vi "Compile - Buffered Tx Channel Refs.vi"(6 "Packet Name":string, 7 "Timestamp Present?":bool, 8 "error in (no error)":errorcluster, 11 "Item Ref in":T1 format="%.0x") -> (0 "error out":errorcluster, 3 "Item Ref out":T1 format="%.0x", 4 "Tx Ref Array":T2(array[cluster]) {"VS Refs" format="%.0x"})   [LabVIEW 2016, in "UDP-Custom-Device System Explorer.lvlib"]
uses:
  UDP-Custom-Device System Explorer.lvlib
  <vilib>/NI Veristand/Custom Device API/Custom Device Item Ref.ctl
  Property Accessors/Tx Packet Accessors.lvlib
  <vilib>/NI VeriStand/Custom Device API/Custom Device API.lvlib
  Property Accessors/Buffered Data Packet.lvlib
  <vilib>/NI VeriStand/Custom Device Tools/Custom Device Utility Library/Custom Device Utility Library.lvlib
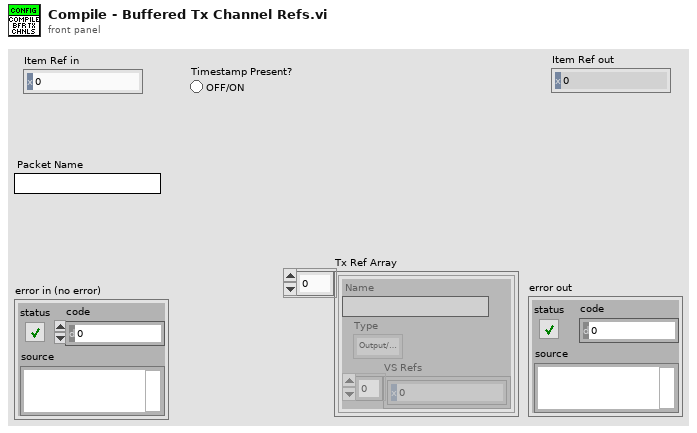
[diagram p1: front panel]
types:
  T1 = typedef "Custom Device API.lvlib/Custom Device Item Ref.ctl" = u64
  T2 = cluster{"Name":string, "Type":enum16{"Output/Write", "Input/Read", "Input/ReadWrite"}, "VS Refs":T1[]}[]
  T3 = enum16{"Output/Write", "Input/Read", "Input/ReadWrite"}
  T4 = cluster{"Name":string, "Type":enum16{"Output/Write", "Input/Read", "Input/ReadWrite"}, "VS Refs":T1[]}
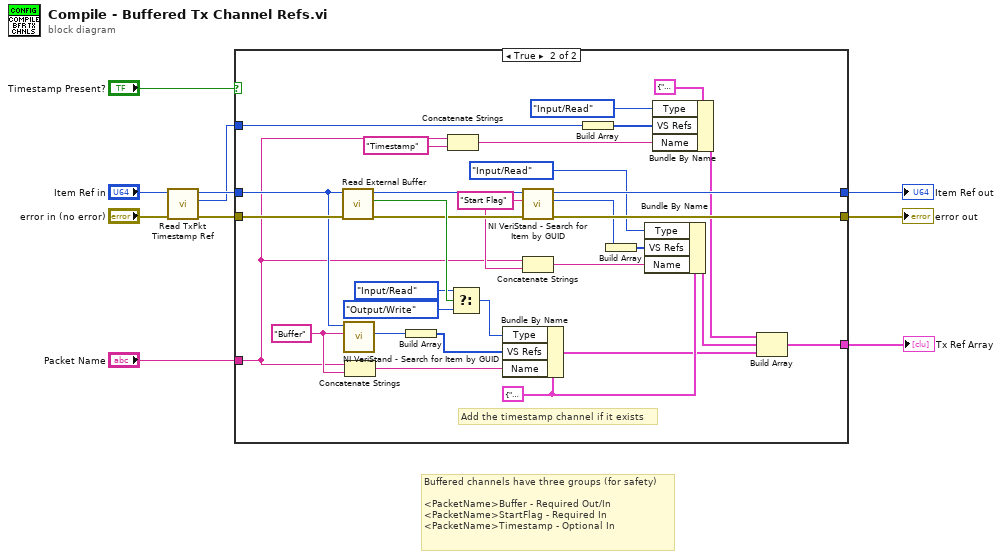
[diagram p0: block diagram]
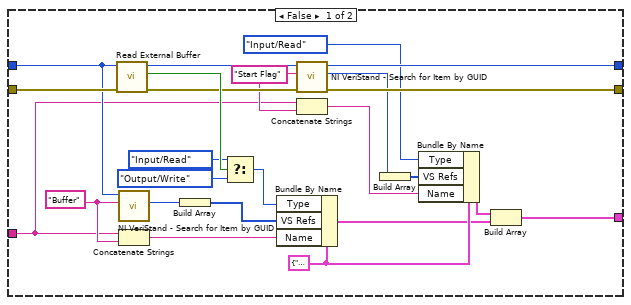
[diagram p2: hidden frame]
diagram:
  # "Buffered channels have three groups (for safety)\n\n<PacketName>Buffer - Required Out/In\n<PacketName>StartFlag - Required In\n<PacketName>Timestamp - Optional In"
  n1 = call "Read TxPkt Timestamp Ref.vi"("error in (no error)"="error in (no error)", "Node Ptr"="Item Ref in") -> ("error out"=w9:errorcluster, "Timestamp Ref"=w8:T1, "Node Ptr out"=w10:T1)  [unwired: 7 in]
  n2 = case shown="True" "Timestamp Present?" {
    tunnel: [w22 w53] -> w2
    tunnel: "Packet Name" -> [w16 w41]
    tunnel: [w11 w43] -> w1
    tunnel: w10 -> [w33 w64]
    tunnel: w9 -> [w34 w65]
    tunnel: w8 -> [_ w38]
    tunnel: [w24 w55] -> w3
    frame False {
      w17 = "Start Flag" ("Item GUID")
      w31 = "Buffer" ("Item GUID")
      w14 = T4 {"Name"="", "Type"=enum."Output/Write", "VS Refs"=[]} ("Group")
      n3 = call "Read External Buffer.vi"("error in (no error)"=w34, "Node Ptr"=w33) -> ("error out"=w23:errorcluster, "External Buffer"=w28:bool, "Node Ptr out"=w25:T1)  [unwired: 7 in]
      n4 = call <vilib>:"NI VeriStand - Search for Item by GUID.vi"("Item GUID"=w31, "Section Ref in"=w33) -> ("Item Ref"=w32:T1)  [unwired: 6 in, 3 out]
      n5 = Concatenate Strings(w16, w31) -> (w30:string)
      n6 = Build Array(w32) -> (w29:T1[])
      n7 = Select(t=T3."Input/Read" ("Type"), s=w28, f=T3."Output/Write" ("Type")) -> (s? t:f=w21:T3)
      n8 = Bundle By Name(cluster=w14, "Type"=w21, "VS Refs"=w29, "Name"=w30) -> (w12:T4)
      n9 = call <vilib>:"NI VeriStand - Search for Item by GUID.vi"("error in"=w23, "Item GUID"=w17, "Section Ref in"=w25) -> ("error out"=w22:errorcluster, "Item Ref"=w19:T1, "Section Ref out"=w24:T1)  [unwired: 5 in, 1 out]
      n10 = Concatenate Strings(w16, w17) -> (w15:string)
      n11 = Build Array(w19) -> (w18:T1[])
      n12 = Bundle By Name(cluster=w14, "Type"=T3."Input/Read", "VS Refs"=w18, "Name"=w15) -> (w13:T4)
      n13 = Build Array(w13, w12) -> (w11:T2)
    }
    frame True {
      w48 = "Start Flag" ("Item GUID")
      w62 = "Buffer" ("Item GUID")
      w46 = T4 {"Name"="", "Type"=enum."Output/Write", "VS Refs"=[]} ("Group")
      # "Add the timestamp channel if it exists"
      n14 = call "Read External Buffer.vi"("error in (no error)"=w65, "Node Ptr"=w64) -> ("error out"=w54:errorcluster, "External Buffer"=w59:bool, "Node Ptr out"=w56:T1)  [unwired: 7 in]
      n15 = call <vilib>:"NI VeriStand - Search for Item by GUID.vi"("Item GUID"=w62, "Section Ref in"=w64) -> ("Item Ref"=w63:T1)  [unwired: 6 in, 3 out]
      n16 = Concatenate Strings(w41, w62) -> (w61:string)
      n17 = Build Array(w63) -> (w60:T1[])
      n18 = Concatenate Strings(w41, "Timestamp" ("Item GUID")) -> (w39:string)
      n19 = Select(t=T3."Input/Read" ("Type"), s=w59, f=T3."Output/Write" ("Type")) -> (s? t:f=w52:T3)
      n20 = Bundle By Name(cluster=w46, "Type"=w52, "VS Refs"=w60, "Name"=w61) -> (w44:T4)
      n21 = call <vilib>:"NI VeriStand - Search for Item by GUID.vi"("error in"=w54, "Item GUID"=w48, "Section Ref in"=w56) -> ("error out"=w53:errorcluster, "Item Ref"=w50:T1, "Section Ref out"=w55:T1)  [unwired: 5 in, 1 out]
      n22 = Concatenate Strings(w41, w48) -> (w47:string)
      n23 = Build Array(w38) -> (w40:T1[])
      n24 = Build Array(w50) -> (w49:T1[])
      n25 = Bundle By Name(cluster=w46, "Type"=T3."Input/Read", "VS Refs"=w49, "Name"=w47) -> (w45:T4)
      n26 = Bundle By Name(cluster=T4 {"Name"="", "Type"=enum."Output/Write", "VS Refs"=[]} ("Group"), "Type"=T3."Input/Read", "VS Refs"=w40, "Name"=w39) -> (w35:T4)
      n27 = Build Array(w35, w45, w44) -> (w43:T2)
    }
  }
  "Tx Ref Array" <- w1
  "error out" <- w2
  "Item Ref out" <- w3
